vi "read_temperature_controller.vi"(2 "Command":string, 3 "delay before read (ms)":u32=75, 4 "VISA resource name":refnum<visa-resource-name>="COM1") -> (0 "Value":string, 1 "Read Buffer":string)   [LabVIEW 2011]
uses:
  <vilib>/Instr/_visa.llb/VISA Configure Serial Port (Instr).vi
panel:
  out "Error Out":errorcluster
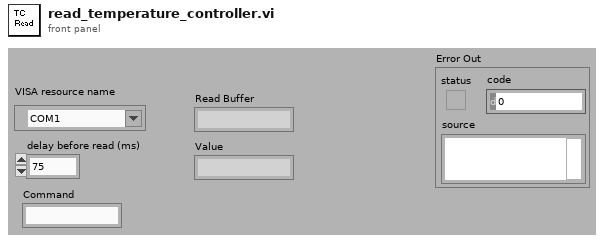
[diagram p1: front panel]
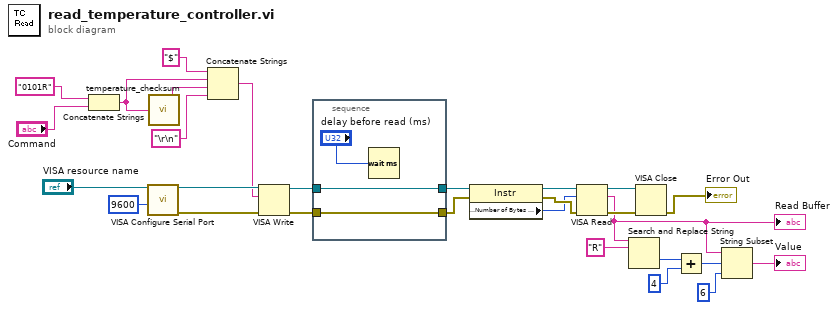
[diagram p0: block diagram]
diagram:
  n1 = Concatenate Strings("0101R" ("write buffer"), "Command") -> (w4:string)
  n2 = call-poly "VISA Configure Serial Port"("VISA resource name"="VISA resource name", "baud rate (9600)"=u32 9600) -> ("VISA resource name out"=w26:refnum<visa-resource-name>, "error out"=w27:errorcluster)  [unwired: 4 in, 8 out]
  n3 = call "temperature_checksum.vi"("Input string"=w4) -> ("Checksum"=w5:string)
  n4 = Concatenate Strings("$" ("string"), w4, w5, "\r\n") -> (w16:string)
  n5 = VISA Write(VISA resource name=w26, write buffer=w16, error in (no error)=w27) -> (VISA resource name out=w21:refnum<visa-resource-name>, error out=w23:errorcluster)  [unwired: 1 out]
  n6 = stacked-sequence {
    tunnel: w23 -> [w31]
    tunnel: [w31] -> w22
    tunnel: w21 -> [w30]
    tunnel: [w30] -> w20
    frame #0 {
      n7 = Wait (ms)(milliseconds to wait="delay before read (ms)") -> ()  [unwired: 1 out]
    }
  }
  n8 = property class="Instr"(reference=w20, error in=w22) -> (reference out=w19:refnum<visa-resource-name>, error out=w18:errorcluster, "Serial Settings:Number of Bytes at Serial Port"=w17:u32)
  n9 = VISA Read(VISA resource name=w19, byte count=w17, error in (no error)=w18) -> (VISA resource name out=w24:refnum<visa-resource-name>, read buffer=w11:string, error out=w25:errorcluster)  [unwired: 1 out]
  "Read Buffer" <- w11
  n10 = Search and Replace String(input string=w11, search string="R") -> (offset past replacement=w13:i32)  [unwired: 1 in, 8 out]
  n11 = VISA Close(VISA resource name=w24, error in (no error)=w25) -> (error out=→"Error Out":errorcluster)
  n12 = Add(x=w13, y=4) -> (x+y=w10:i32)
  n13 = String Subset(string=w11, offset (0)=w10, length (rest)=6 ("length (rest)")) -> (substring=→"Value":string)
